vi "PH_GetSwitchInformation.get and prepare Info.vi"(5 "error in":errorcluster) -> (14 "ColHdrs[]":string[](array[string])=["Sixpack Instance", "Axis"], 15 "RowHdrs[]":string[](array[string]), 16 "ItemNames":string[][](array[string]), 17 "Row Cell BG":u32[](array[numeric]), 19 "error out":errorcluster)   [LabVIEW 2014, in "PH_GetSwitchInformation.lvlib"]
doc: "This VI is reading out information from the database and prepares it for the visualisation on the GUI."
uses:
  PH_GetSwitchInformation.lvlib
  PH_Common/PH_Common.lvlib
  CSCore/CSSystem/CSSystemLib/CSSystemLib.lvlib
  PH_PSDBWriter/PH_PSDBWriter.lvlib
  PH_Switch/PH_Switch.lvlib
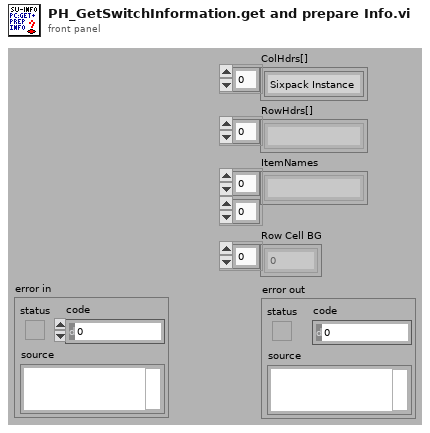
[diagram p1: front panel]
types:
  T1 = cluster{"Switch":string, "True":string, "False":string}
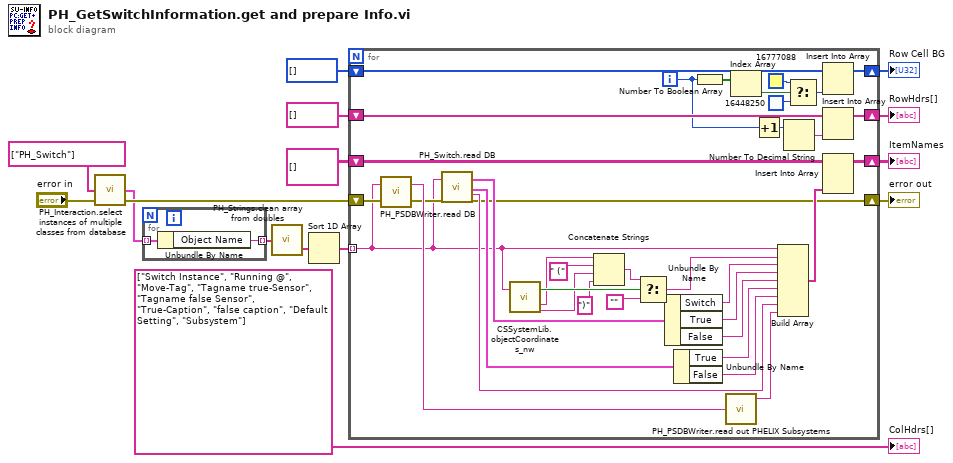
[diagram p0: block diagram]
diagram:
  n1 = call "PH_Interaction.select instances of multiple classes from database.vi"("error in (no error)"="error in", "Classes Input"=string[] ["PH_Switch"]) -> ("error out"=w5:errorcluster, "Query Result"=w4:cluster{"Object Name":string, "Class":string}[])  [unwired: 2 in]
  n2 = for {
    tunnel: w4 -> [w17] mode=indexing
    tunnel: [w16] -> w3 mode=indexing
    n3 = Unbundle By Name(w17) -> ("Object Name"=w16:string)
  }
  n4 = call "PH_Strings.clean array from doubles.vi"("Array Input"=w3) -> ("Cleaned Array Output"=w2:string[])  [unwired: 1 out]
  n5 = Sort 1D Array(array=w2) -> (sorted array=w1:string[])
  n6 = for {
    tunnel: w1 -> [w18] mode=indexing
    shift-right: [w54] -> w10
    shift-left: string[][] [] -> [w53]
    shift-right: [w50] -> w12
    shift-left: string[] [] -> [w51]
    shift-right: [w48] -> w14
    shift-left: u32[] [] -> [w47]
    shift-right: [w19] -> w15
    shift-left: w5 -> [w30]
    i -> [w37]
    n7 = call "PH_PSDBWriter.read DB.vi"("error in"=w30, "Instance Name"=w18) -> ("error out"=w28:errorcluster, "PSDB Subsystem"=w29:string)
    n8 = call "PH_Switch.read DB.vi"("DB Entry to read"=w18, "error in (no error)"=w28) -> ("Tagnames"=w27:T1, "Captions"=w22:cluster{"True":string, "False":string}, "Default Value"=w23:string, "error out"=w19:errorcluster)  [unwired: 13 in, 1 out]
    n9 = call "CSSystemLib.objectCoordinates_nw.vi"("name"=w18) -> ("obj exists"=w46:bool, "systemID"=w43:string, "node"=w40:string)  [unwired: 15 in, 1 out]
    n10 = Concatenate Strings(w43, " (" ("string"), w40, ")" ("string")) -> (w42:string)
    n11 = Select(t=w42, s=w46, f="") -> (s? t:f=w44:string)
    n12 = Unbundle By Name(w27) -> ("Switch"=w26:string, "True"=w25:string, "False"=w24:string)
    n13 = Unbundle By Name(w22) -> ("True"=w21:string, "False"=w20:string)
    n14 = Number To Boolean Array(number=w37) -> (Boolean array=w34:bool[])
    n15 = call "PH_PSDBWriter.read out PHELIX Subsystems.vi"("Config DB Subsystem"=w29) -> ("Subsystem"=w31:string)  [unwired: 2 in, 2 out]
    n16 = Index Array(array=w34) -> (element=w35:bool)  [unwired: 1 in]
    n17 = Increment(x=w37) -> (x+1=w36:i32)
    n18 = Build Array(w18, w44, w26, w25, w24, w21, w20, w23, w31) -> (w38:string[])
    n19 = Number To Decimal String(number=w36) -> (decimal integer string=w52:string)  [unwired: 1 in]
    n20 = Select(t=u32 16777088 ("Color Box"), s=w35, f=u32 16448250 ("Color Box")) -> (s? t:f=w49:u32)
    n21 = Insert Into Array(array=w47, new element=w49) -> (w48:u32[])  [unwired: 1 in]
    n22 = Insert Into Array(array=w51, new element=w52) -> (w50:string[])  [unwired: 1 in]
    n23 = Insert Into Array(array=w53, new element=w38) -> (w54:string[][])  [unwired: 2 in]
  }
  "error out" <- w15
  "Row Cell BG" <- w14
  "RowHdrs[]" <- w12
  "ItemNames" <- w10
  "ColHdrs[]" <- string[] ["Switch Instance", "Running @", "Move-Tag", "Tagname true-Sensor", "Tagname false Sensor", "True-Caption", "false caption", "Default Setting", "Subsystem"] ("new element/subarray")
